vi "Write Averaging time.vi"(8 "error in (no error)":errorcluster, 10 "Averaging time":dbl, 11 "Write Averaging time Msg in":refnum<class "Write Averaging time Msg.lvclass">) -> (0 "error out":errorcluster, 3 "Write Averaging time Msg out":refnum<class "Write Averaging time Msg.lvclass">)   [LabVIEW 2015, in "Write Averaging time Msg.lvclass"]
uses:
  Write Averaging time Msg.lvclass
  Write Averaging time Msg.lvclass/Write Averaging time Msg.ctl
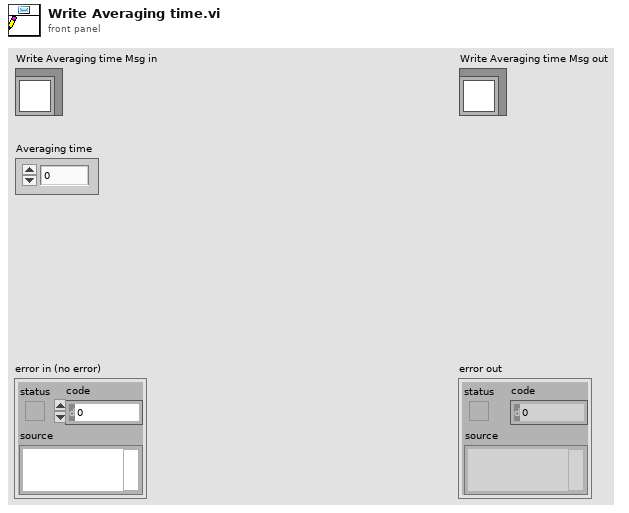
[diagram p1: front panel]
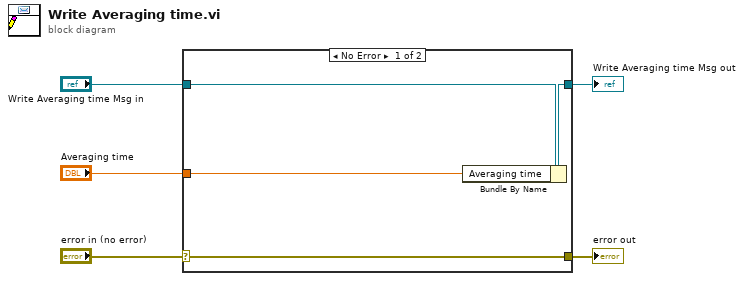
[diagram p0: block diagram]
diagram:
  n1 = case shown="No Error" "error in (no error)" {
    selector: "error in (no error)" -> [w9 w10]
    tunnel: [w9 w10] -> w4
    tunnel: [w7 w11] -> w2
    tunnel: "Write Averaging time Msg in" -> [w8 w11]
    tunnel: "Averaging time" -> [w6 _]
    frame No Error {
      n2 = Bundle By Name(cluster=w8, "Averaging time"=w6) -> (w7:refnum<class "Write Averaging time Msg.lvclass">)
    }
    frame Error {
    }
  }
  "error out" <- w4
  "Write Averaging time Msg out" <- w2
